vi "Try Decimal Value.vi"(6 "Negate?":bool, 8 "error in (no error)":errorcluster, 10 "Scaling Info":T1={"Bit Offset"=0, "Bit Count"=0, "LSB Resolution"=0.1, "2's Complement"=FALSE, "Big Endian"=FALSE, "Sign Bit"=FALSE}, 11 "Random Attempts":i32=100) -> (0 "error out":errorcluster)   [LabVIEW 2020, in "Unit Tests.lvlib" / "Data Scaling.lvclass"]
uses:
  Data Scaling.lvclass
  Frames & Messages/TypeDefs/Scaling Information.ctl
  <vilib>/addons/_JKI Toolkits/Caraya/classes/Assert/Assert.lvclass
  BCI-1553 API.lvlib
panel:
  in  "Override":bool
  in  "Override Value":dbl=-20.0 format="%#_13g"
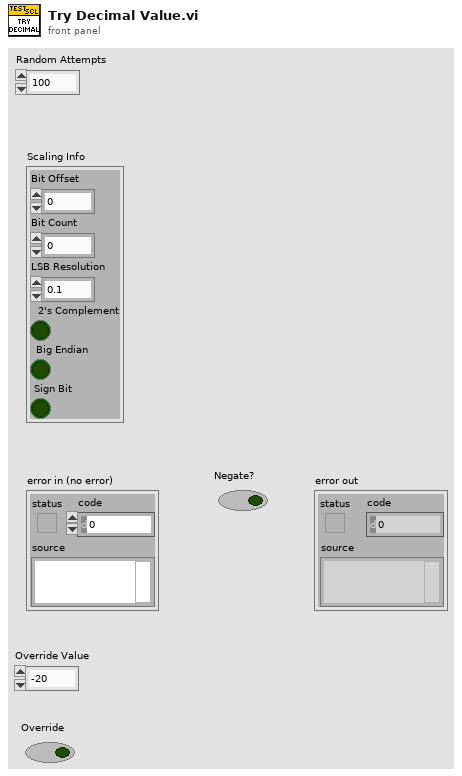
[diagram p1: front panel]
types:
  T1 = typedef "BCI-1553 API.lvlib/Scaling Information.ctl" = cluster{"Bit Offset":i32, "Bit Count":i32, "LSB Resolution":dbl, "2's Complement":bool, "Big Endian":bool, "Sign Bit":bool}
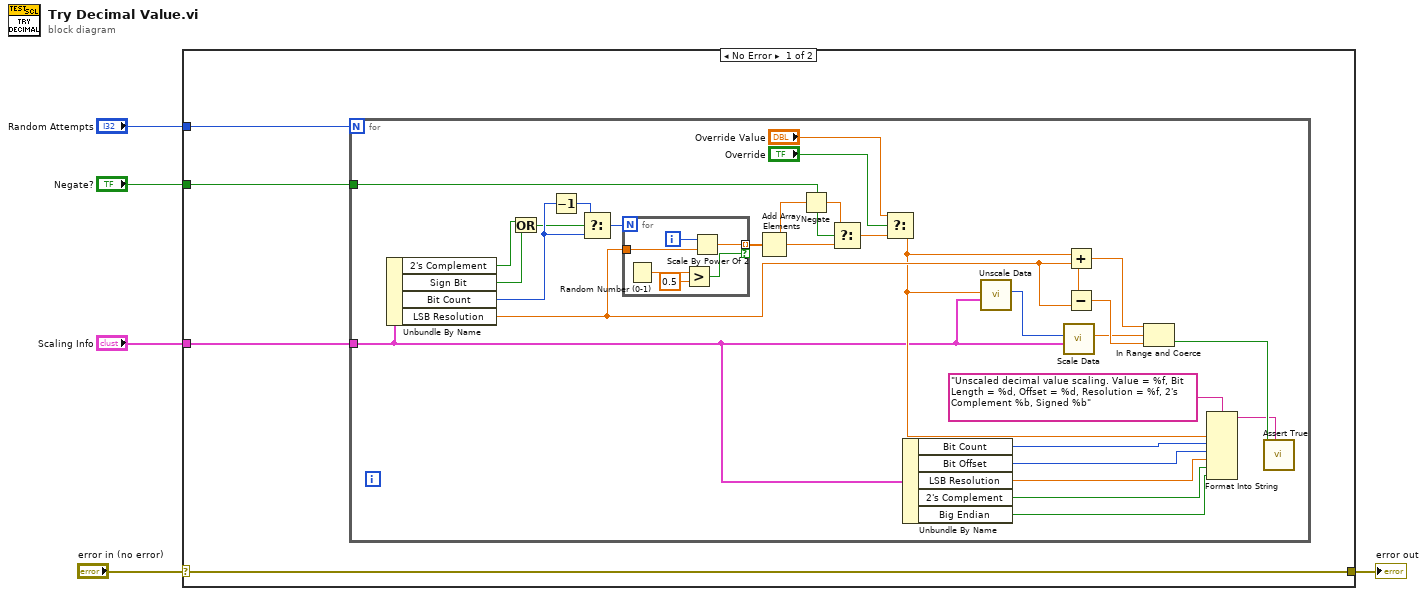
[diagram p0: block diagram]
diagram:
  n1 = case shown="No Error" "error in (no error)" {
    selector: "error in (no error)" -> [w9 w44]
    tunnel: [w9 w44] -> w4
    tunnel: "Random Attempts" -> [w8 _]
    tunnel: "Scaling Info" -> [w6 _]
    tunnel: "Negate?" -> [w7 _]
    frame No Error {
      n2 = for {
        N: w8 -> [_]
        tunnel: w6 -> [w11]
        tunnel: w7 -> [w17]
        n3 = Unbundle By Name(w11) -> ("2's Complement"=w16:bool, "Sign Bit"=w19:bool, "Bit Count"=w21:i32, "LSB Resolution"=w33:dbl)
        n4 = Or(x=w16, y=w19) -> (x .or. y?=w18:bool)
        n5 = Decrement(x=w21) -> (x-1=w22:i32)
        n6 = Select(t=w22, s=w18, f=w21) -> (s? t:f=w20:i32)
        n7 = for {
          N: w20 -> [_]
          tunnel: w33 -> [w38]
          tunnel: [w42] -> w34 mode=indexing if=w39
          i -> [w43]
          n8 = Random Number (0-1)() -> (number: 0 to 1=w41:dbl)
          n9 = Greater?(x=w41, y=0.5) -> (0:w39:bool)
          n10 = Scale By Power Of 2(n=w43, x=w38) -> (x*2^n=w42:dbl)
        }
        n11 = Add Array Elements(numeric array=w34) -> (sum=w26:dbl)
        n12 = Negate(x=w26) -> (-x=w27:dbl)
        n13 = Select(t=w27, s=w17, f=w26) -> (s? t:f=w25:dbl)
        n14 = Select(t="Override Value", s="Override", f=w25) -> (s? t:f=w13:dbl)
        n15 = Unbundle By Name(w11) -> ("Bit Count"=w30:i32, "Bit Offset"=w31:i32, "LSB Resolution"=w32:dbl, "2's Complement"=w15:bool, "Big Endian"=w14:bool)
        n16 = call "Unscale Data.vi"("Scaling Info"=w11, "Scaled Value"=w13) -> ("Raw Value"=w10:u64)  [unwired: 8 in, 1 out]
        n17 = call "Scale Data.vi"("Scaling Info"=w11, "Raw Value"=w10) -> ("Scaled Value"=w12:dbl)  [unwired: 8 in, 1 out]
        n18 = Add(x=w13, y=w33) -> (x+y=w37:dbl)
        n19 = Subtract(x=w13, y=w33) -> (x-y=w36:dbl)
        n20 = In Range and Coerce(upper limit=w37, x=w12, lower limit=w36) -> (In Range?=w35:bool)  [unwired: 1 out]
        n21 = Format Into String(format string="Unscaled decimal value scaling. Value = %f, Bit Length = %d, Offset = %d, Resolution = %f, 2's Complement %b, Signed %b" ("Label"), w13, w30, w31, w32, w15, w14) -> (resulting string=w28:string)  [unwired: 2 in, 1 out]
        n22 = call <vilib>:"Assert True.vi"("Label"=w28, "True?"=w35) -> ()  [unwired: 8 in, 2 out]
      }
    }
    frame Error {
    }
  }
  "error out" <- w4
